vi "Main VI.vi"() -> ()   [LabVIEW 2022 SP3]
uses:
  <vilib>/National Instruments/NIPM API (Beta)/NIPM_API.lvlib
  NIPM_Functions/NIPM_Functions.lvlib
panel:
  in  "SelfUpgrade":bool
  out "Upgradable":bool
  out "Last Version Available":string
  out "Package Installed Version":string
  out "versions":string[](array[string])
  in  "Upgrade?":bool
  in  "AvailableVersions":bool
  out "Time":timestamp format="%<%x %.0X>T"
  out "Application Version":string
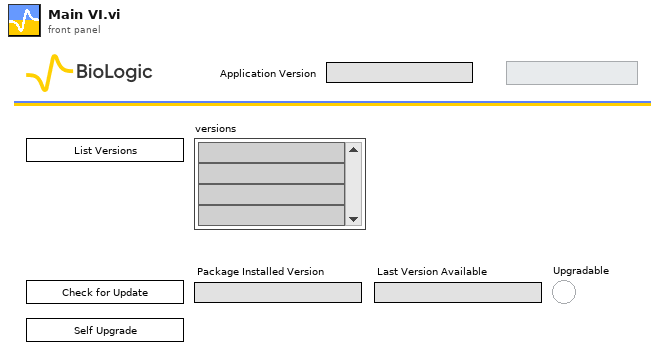
[diagram p1: front panel]
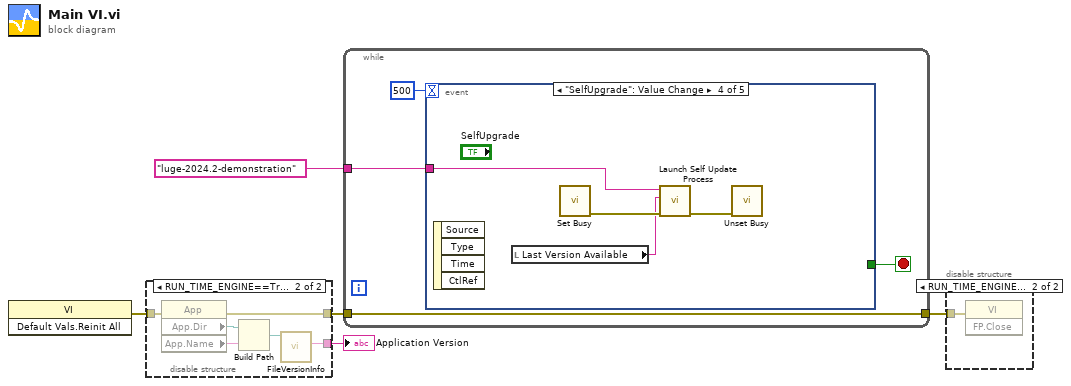
[diagram p0: block diagram]
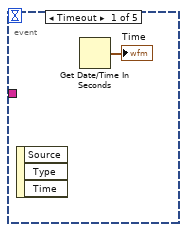
[diagram p3: hidden frame]
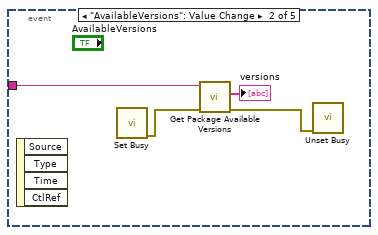
[diagram p4: hidden frame]
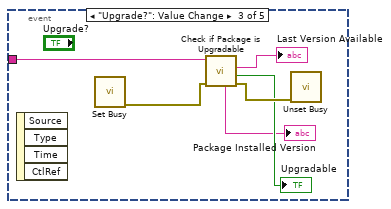
[diagram p5: hidden frame]
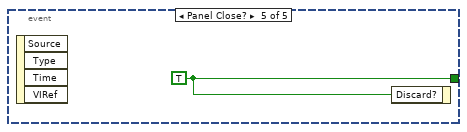
[diagram p6: hidden frame]
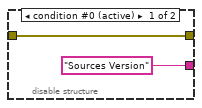
[diagram p7: hidden frame]
diagram:
  n1 = invoke class="VI" method="Default Vals.Reinit All"() -> (error out=w1:errorcluster)  [unwired: 3 in, 2 out]
  n2 = disable-structure shown="RUN_TIME_ENGINE==True" {
    disable-tunnel: ["Sources Version" ("Application Version") w13] -> w5
    disable-tunnel: [w6 w9] -> w4
    disable-tunnel: w1 -> [w6 w8]
    frame condition #0 (active) {
    }
    frame condition #1 {
      n3 = property class="App"(error in=w8) -> (error out=w9:errorcluster, "App.Dir"=w12:path, "App.Name"=w11:string)  [unwired: 1 in, 1 out]
      n4 = Build Path(base path=w12, name or relative path=w11) -> (appended path=w10:path)
      n5 = call <vilib>:"FileVersionInfo.vi"("Application Path in"=w10) -> ("File Version Info"=w13:string)  [unwired: 7 in, 3 out]
    }
  }
  "Application Version" <- w5
  n6 = while {
    tunnel: w4 -> [w15]
    tunnel: [w15] -> w3
    tunnel: "luge-2024.2-demonstration" -> [w14]
    stop <- w16 stop-if-true
    n7 = event shown="[3] \"SelfUpgrade\": Value Change" {
      selector: _ -> [_ _ _ _ _]
      dyn-events: _ -> [_ _ _ _ _]
      timeout: 500 -> [_ _ _ _ _]
      tunnel: [_ _ _ _ w33] -> w16
      tunnel: w14 -> [_ w22 w27 w32 _]
      event Timeout {
        n8 = event-data() -> ()  [unwired: 1 in, 3 out]
        n9 = Get Date/Time In Seconds() -> (seconds since 1Jan1904=→"Time":timestamp)
      }
      event "AvailableVersions": Value Change {
        n10 = event-data() -> ()  [unwired: 1 in, 4 out]
        n11 = call <vilib>:"Set Busy.vi"() -> ("error out"=w20:errorcluster)  [unwired: 10 in, 1 out]
        n12 = call <vilib>:"Get Package Available Versions.vi"("error in"=w20, "package name"=w22) -> ("error out"=w19:errorcluster, "versions"=→"versions":string[])  [unwired: 7 in, 1 out]
        n13 = call <vilib>:"Unset Busy.vi"("error in (no error)"=w19) -> ()  [unwired: 10 in, 1 out]
      }
      event "Upgrade?": Value Change {
        n14 = event-data() -> ()  [unwired: 1 in, 4 out]
        n15 = call <vilib>:"Set Busy.vi"() -> ("error out"=w28:errorcluster)  [unwired: 10 in, 1 out]
        n16 = call <vilib>:"Check if Package is Upgradable.vi"("error in"=w28, "package name"=w27) -> ("error out"=w26:errorcluster, "upgradable?"=→"Upgradable":bool, "version to upgrade to"=→"Last Version Available":string, "currently installed version"=→"Package Installed Version":string)  [unwired: 5 in, 1 out]
        n17 = call <vilib>:"Unset Busy.vi"("error in (no error)"=w26) -> ()  [unwired: 10 in, 1 out]
      }
      event "SelfUpgrade": Value Change {
        n18 = event-data() -> ()  [unwired: 1 in, 4 out]
        n19 = local read "Last Version Available"() -> (w29:string)
        n20 = call <vilib>:"Set Busy.vi"() -> ("error out"=w31:errorcluster)  [unwired: 10 in, 1 out]
        n21 = call "Launch Self Update Process.vi"("error in (no error)"=w31, "Version"=w29, "Package Name"=w32) -> ("error out"=w30:errorcluster)  [unwired: 8 in]
        n22 = call <vilib>:"Unset Busy.vi"("error in (no error)"=w30) -> ()  [unwired: 10 in, 1 out]
      }
      event Panel Close? {
        w33 = TRUE ("Discard?")
        n23 = event-data() -> ()  [unwired: 1 in, 4 out]
        n24 = event-data("Discard?"=w33) -> ()  [unwired: 1 in, 1 out]
      }
    }
  }
  n25 = disable-structure shown="RUN_TIME_ENGINE==True" {
    disable-tunnel: w3 -> [_ w34]
    frame condition #0 (active) {
    }
    frame condition #1 {
      n26 = invoke class="VI" method="FP.Close"(error in=w34) -> ()  [unwired: 2 in, 3 out]
    }
  }
